vi "force_control_globals.vi"() -> ()   [LabVIEW 2013]
uses:
  <vilib>/Analysis/Matrix/Datatypes/RealMatrix.ctl
  <vilib>/Analysis/Matrix/NI_Matrix.lvlib
panel:
  in  "Y Ki Degradation":dbl=0.005
  in  "force_injection_Z":T1(ring)
  in  "force_controlType_Z":T2(ring)=enum."One Way Threshold"
  in  "force_injection_Y":T1(ring)
  in  "force_controlType_Y":T2(ring)=enum."One Way Threshold"
  in  "force_injection_X":T1(ring)
  in  "force_controlType_X":T2(ring)=enum."One Way Threshold"
  in  "X Ki Degradation":dbl=0.0025
  in  "Reset":bool
  in  "Ka Slope Limit":i32=6
  in  "Ka Gains":sgl[](array[numeric])=[0.7, 0.0, 0.0] format="%#_6p"
  in  "Error Threshold":sgl[](array[numeric])=[0.3, 0.3, 0.3] format="%#_6p"
  in  "Force Threshold":sgl[](array[numeric])=[0.0, 0.3, 0.3] format="%#_6p"
  in  "Force Control":bool
  in  "Inject Stimulus":bool
  in  "Override with Stimulus":bool
  in  "Force Stimulus":dbl[](array[numeric])=[0.0, 0.0, 0.0]
  in  "Control Axis":bool[](array[boolean])=[FALSE, FALSE, TRUE]
  in  "Force Max Acceleration":i32=2
  in  "Force Max Speed":i32=10
  in  "Hard Threshold":sgl[](array[numeric])=[0.0, 8.0, 12.0] format="%#_6p"
  in  "Soft Threshold":sgl[](array[numeric])=[5.0, 5.0, 8.0] format="%#_6p"
  in  "Kd Slope Limit":i32=6
  in  "PseudoInv Force Calibration":dbl[][](array[numeric])=[[121.8841, 55.8527, -16.4824], [92.1962, 156.6746, 43.823]]
  in  "Force Calibration":dbl[][](array[numeric])
  in  "Granularity":dbl=1000000.0
  in  "Maximum Translation":i32=3000
  in  "Kd Gains":sgl[](array[numeric])=[0.04, 0.01, 0.0] format="%#_6p"
  in  "Ki Gains":sgl[](array[numeric])=[1.0, 0.8, 0.6] format="%#_6p"
  in  "Kp Gains":sgl[](array[numeric])=[1.4, 1.4, 1.4] format="%#_6p"
  in  "Surface Vector Input":enum16{"Accelerometer", "Plane Normal"}(ring)
  in  "ASAP to Surface Rotation Matrix":T3=[[-0.94340685160565, -0.32848364418107, 0.045629024195576, 9068.109203025148], [0.283835534373385, -0.870906704437691, -0.401196836468652, -24863.68471797479], [0.171525221966017, -0.365540705901551, 0.914854682754865, -63368.71671959403], [0.0, 0.0, 0.0, 1.0]]
  # "Force Control Type"
  # "Force Injection Type"
  # "X Axis"
  # "Y Axis"
  # "Z Axis"
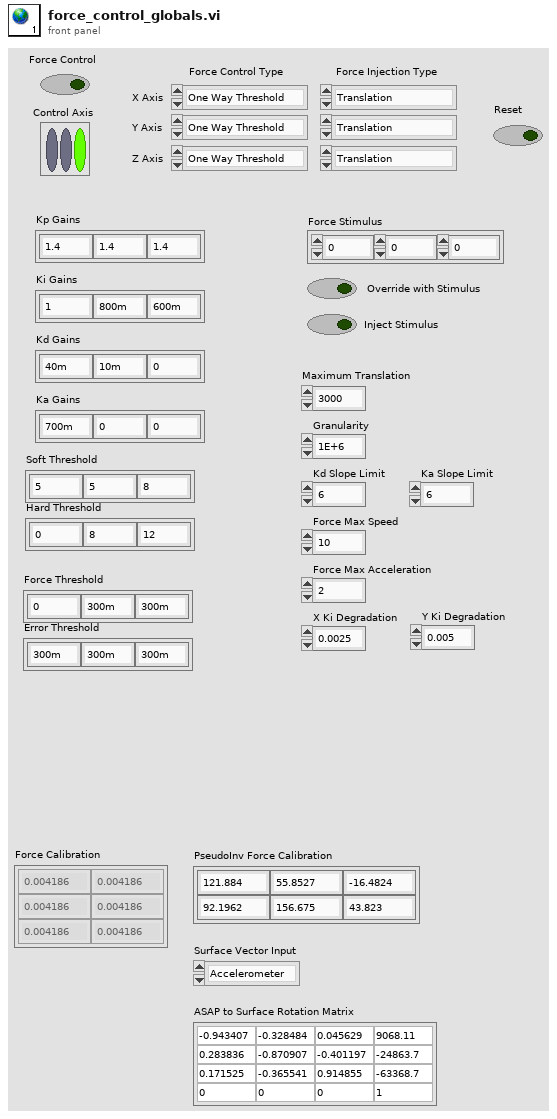
[diagram p1: front panel]
types:
  T1 = enum16{"Translation", "Tip Position", "Rotation"}
  T2 = enum16{"Setpoint", "One Way Threshold", "Two Way Threshold"}
  T3 = typedef "NI_Matrix.lvlib/RealMatrix.ctl" = dbl[][]
diagram:
